vi "upper case and lower case string.vi"() -> ()   [LabVIEW 2025]
panel:
  out "lower case":string
  out "output string upper case":string
  in  "input string":string
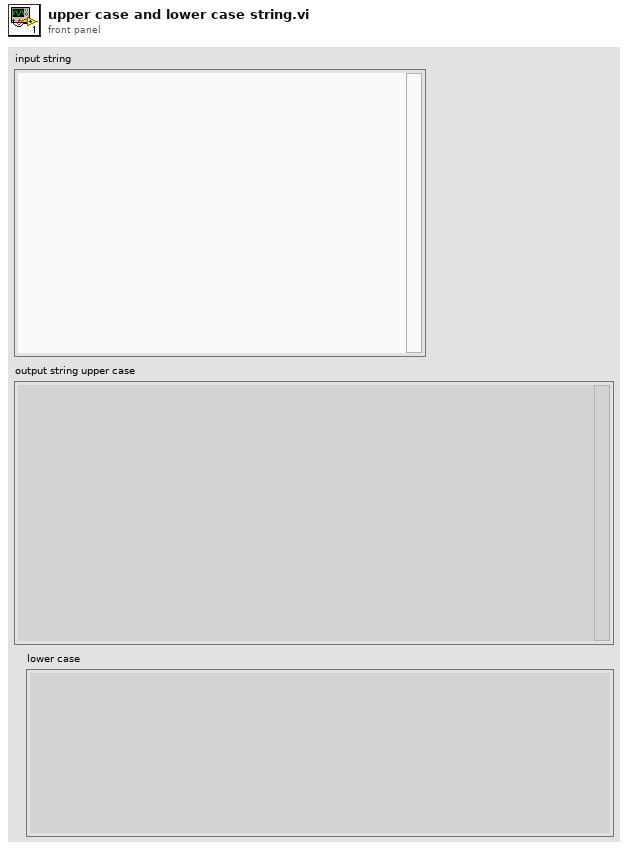
[diagram p1: front panel]
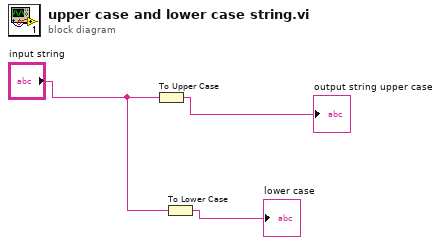
[diagram p0: block diagram]
diagram:
  n1 = To Upper Case(1:"input string") -> (0:→"output string upper case":string)
  n2 = To Lower Case(string="input string") -> (all lower case string=→"lower case":string)
